vi "Filter Log Packet.vi"(10 "Log Packet":T1, 11 "Event Level Filter in":refnum<class "Event Level Filter.lvclass">) -> (2 "Log?":bool, 3 "Event Level Filter out":refnum<class "Event Level Filter.lvclass">)   [LabVIEW 2020, in "Event Level Filter.lvclass"]
uses:
  <vilib>/gpm_packages/@cs/event-logger/Source/Filters/Event Level Filter/Event Level Filter.lvclass
  <vilib>/gpm_packages/@cs/event-logger/Source/Composed Log/Types/Log Packet.ctl
  <vilib>/gpm_packages/@cs/event-logger/Source/Composed Log/Types/Log Level.ctl
  <vilib>/gpm_packages/@cs/event-logger/Source/Filters/Event Level Filter/Event Level Filter.lvclass/Event Level Filter.ctl
  <vilib>/gpm_packages/@cs/event-logger/Source/Composed Log/Composed Log.lvlib
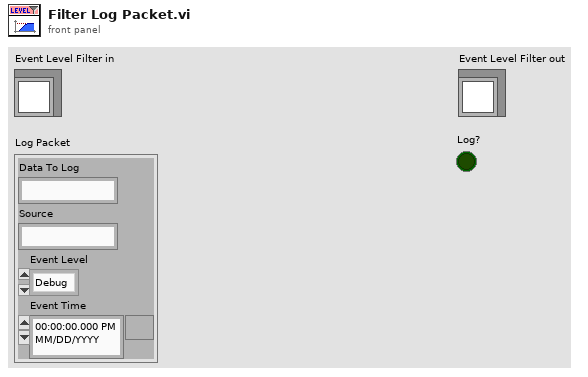
[diagram p1: front panel]
types:
  T1 = typedef "Composed Log.lvlib/Log Packet.ctl" = cluster{"Data To Log":string, "Source":string, "Event Level":T2, "Event Time":timestamp}
  T2 = typedef "Composed Log.lvlib/Log Level.ctl" = enum16{"Debug", "Info", "Warning", "Error", "Critical"}
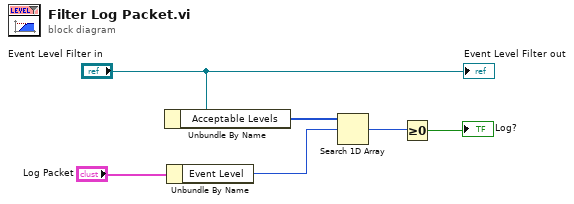
[diagram p0: block diagram]
diagram:
  n1 = Unbundle By Name("Event Level Filter in") -> ("Acceptable Levels"=w4:T2[])
  n2 = Unbundle By Name("Log Packet") -> ("Event Level"=w3:T2)
  n3 = Search 1D Array(1D array=w4, element=w3) -> (index of element=w2:i32)  [unwired: 1 in]
  n4 = Greater Or Equal To 0?(x=w2) -> (x >= 0?=→"Log?":bool)
  "Event Level Filter out" <- "Event Level Filter in"
